vi "Counter.vi"() -> (2 "Counter":dbl)   [LabVIEW 2015]
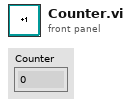
[diagram p1: front panel]
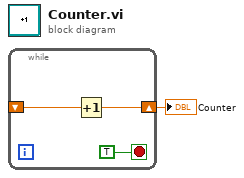
[diagram p0: block diagram]
diagram:
  n1 = while {
    shift-right: [w3] -> w1
    shift-left: _ -> [w2]
    stop <- TRUE stop-if-true
    n2 = Increment(x=w2) -> (x+1=w3:dbl)
  }
  "Counter" <- w1
